vi "ECG heart rate calculation.vi"() -> ()   [LabVIEW 2024]
uses:
  <vilib>/Utility/file.llb/Read Delimited Spreadsheet (DBL).vi
  <vilib>/Analysis/NI_AAL_SigProc.lvlib
panel:
  out "Techyardik\n 2":bool
  out "brady 2":bool
  out "S.R 2":bool
  out "Heartrate (bpm) 2":i32
  out "BPM":dbl
  in  "samplinng Rate":i32
  out "Heartrate (bpm)":i32
  out "S.R":bool
  out "brady":bool
  out "Techyardik":bool
  in  "threshold":dbl format="%0.2f"
  in  "stop":bool
  out "size(s) 2":i32
  out "subarray 2":dbl[](array[numeric])
  out "subarray":dbl[](array[numeric])
  out "XY Graph":cluster{"all rows":dbl[], "all rows":dbl[]}(graph)
  out "all rows":dbl[][](array[numeric])
  in  "file path (dialog if empty)":path
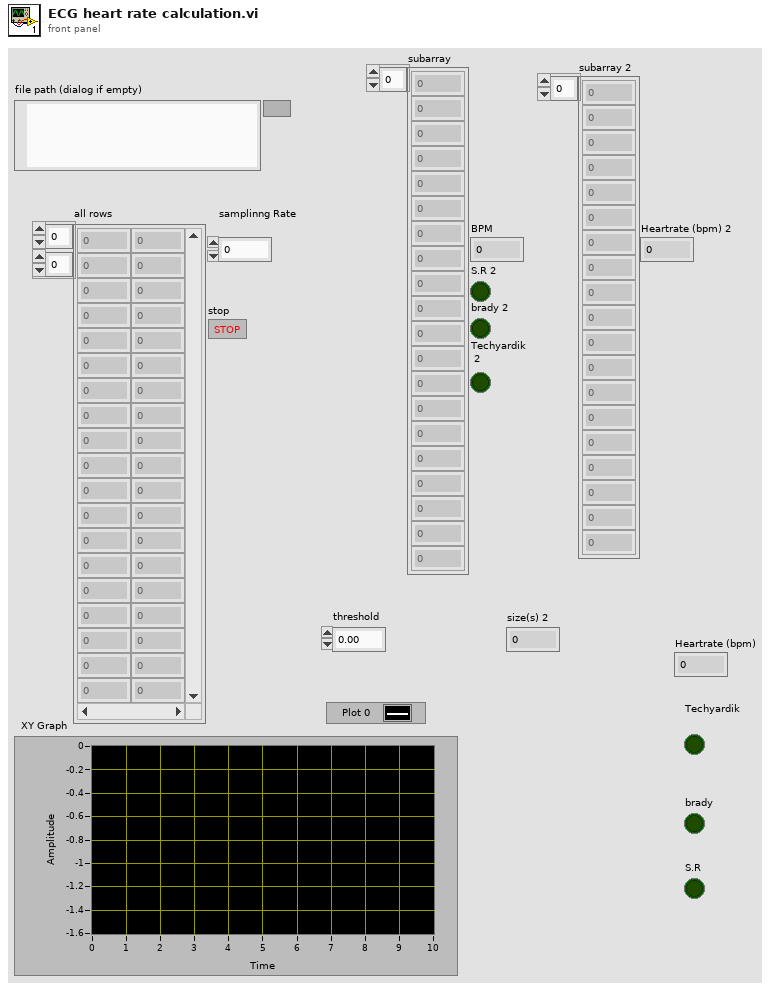
[diagram p1: front panel]
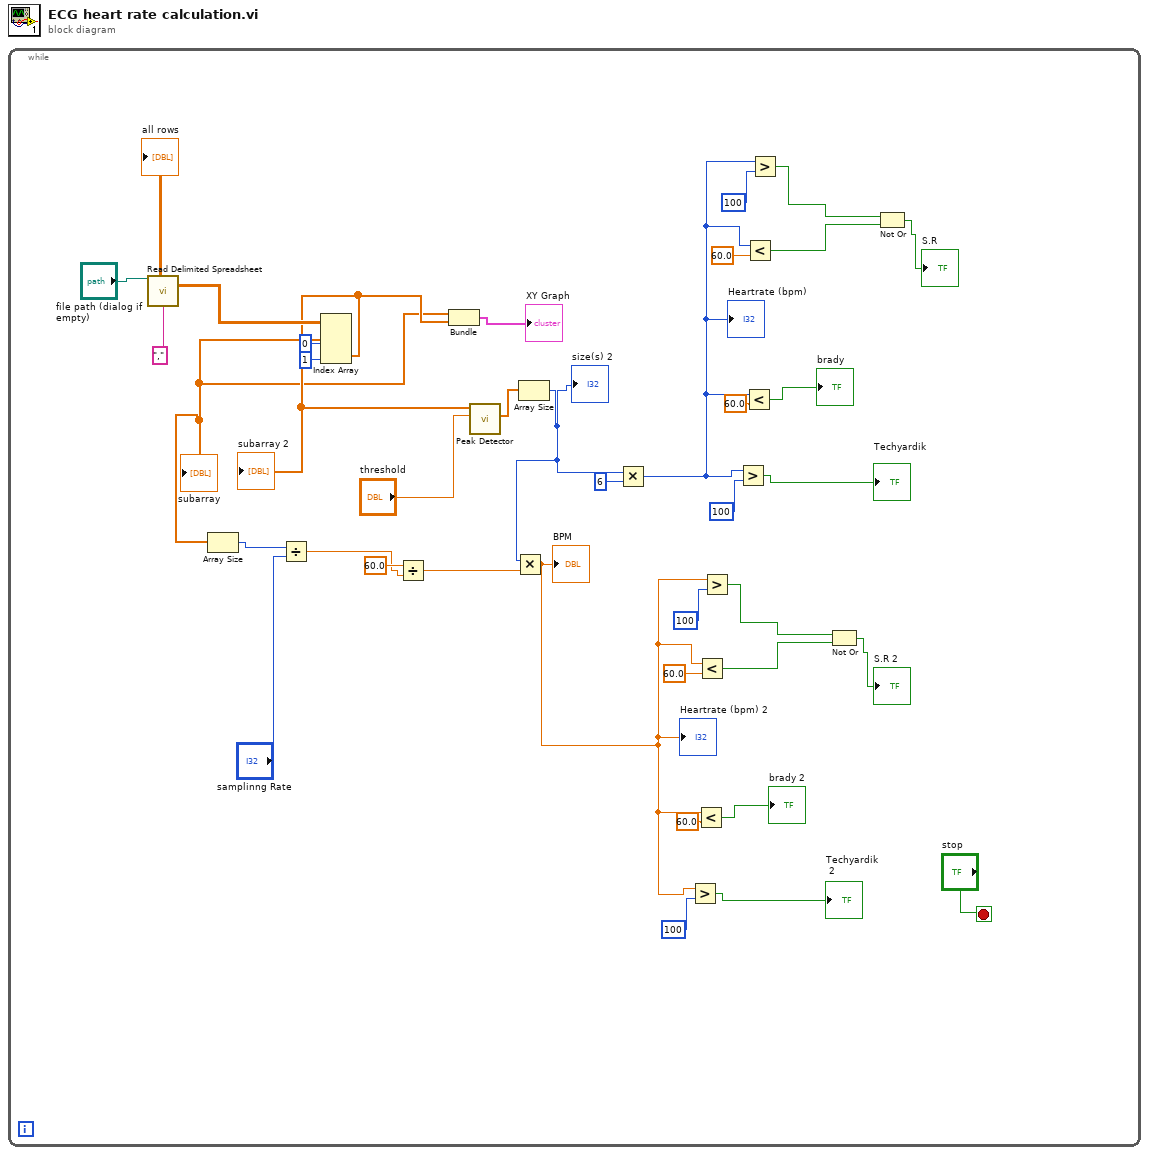
[diagram p0: block diagram]
diagram:
  n1 = while {
    stop <- "stop" stop-if-true
    n2 = call-poly <vilib>:"Read Delimited Spreadsheet.vi"("file path (dialog if empty)"="file path (dialog if empty)", "delimiter (\\t)"="," ("delimiter (\\t)")) -> ("all rows"=w36:dbl[][])  [unwired: 8 in, 5 out]
    "all rows" <- w36
    n3 = Index Array(array=w36, index (col) #1=0 ("disabled index (col)"), index (col) #2=1 ("index (col)")) -> (element #1=w20:dbl[], element #2=w31:dbl[])  [unwired: 2 in]
    "subarray" <- w20
    "subarray 2" <- w31
    n4 = Array Size(array=w20) -> (size(s)=w19:i32)
    n5 = Divide(x=w19, y="samplinng Rate") -> (x/y=w16:dbl)
    n6 = Divide(x=60.0, y=w16) -> (x/y=w15:dbl)
    n7 = Bundle("all rows"=w20, "all rows"=w31) -> (→"XY Graph":cluster{"all rows":dbl[], "all rows":dbl[]})  [unwired: 1 in]
    n8 = call <vilib>:"Peak Detector.vi"("threshold"="threshold", "X"=w31) -> ("Amplitudes"=w32:dbl[])  [unwired: 5 in, 4 out]
    n9 = Array Size(array=w32) -> (size(s)=w14:i32)
    "size(s) 2" <- w14
    n10 = Multiply(x=w14, y=w15) -> (x*y=w1:dbl)
    "BPM" <- w1
    "Heartrate (bpm) 2" <- w1
    n11 = Multiply(x=w14, y=6) -> (x*y=w21:i32)
    "Heartrate (bpm)" <- w21
    n12 = Greater?(x=w1, y=100) -> (0:→"Techyardik\n 2":bool)
    n13 = Less?(x=w1, y=60.0) -> (x < y?=→"brady 2":bool)
    n14 = Less?(x=w1, y=60.0) -> (x < y?=w9:bool)
    n15 = Greater?(x=w1, y=100) -> (0:w8:bool)
    n16 = Greater?(x=w21, y=100) -> (0:→"Techyardik":bool)
    n17 = Less?(x=w21, y=60.0) -> (x < y?=→"brady":bool)
    n18 = Less?(x=w21, y=60.0) -> (x < y?=w12:bool)
    n19 = Greater?(x=w21, y=100) -> (0:w13:bool)
    n20 = Not Or(1:w9, 2:w8) -> (0:→"S.R 2":bool)
    n21 = Not Or(1:w12, 2:w13) -> (0:→"S.R":bool)
  }
